vi "XNET.Cluster.Stream.Initialize.vi"(8 "error in":errorcluster, 10 "CAN Cluster":T1={"64bit Baud Rate"=125000, "Comment"="", "Name"="", "Transmit I/O Mode"=0, "64bit FD Baud Rate"=0} {"Transmit I/O Mode" items=["CAN 2.0", "CAN FD", "CAN FD+BRS"]}, 11 "database in":refnum<k21>) -> (0 "error out":errorcluster, 3 "cluster out":refnum<k21>)   [LabVIEW 2019, in "Diagnostics Addon Engine.lvlib"]
uses:
  Types/XNET.Cluster.ctl
  Diagnostics Addon Engine.lvlib
  <vilib>/xnet/xnet.llb/XNET Database Create (Cluster).vi
  <resource>/objmgr/xnet.rc
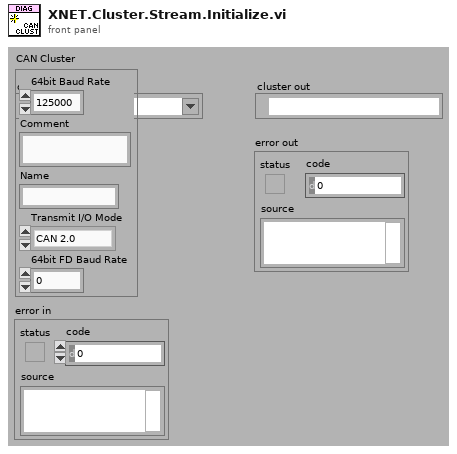
[diagram p1: front panel]
types:
  T1 = typedef "Diagnostics Addon Engine.lvlib/XNET.Cluster.ctl" = cluster{"64bit Baud Rate":u64, "Comment":string, "Name":string, "Transmit I/O Mode":u32, "64bit FD Baud Rate":u64}
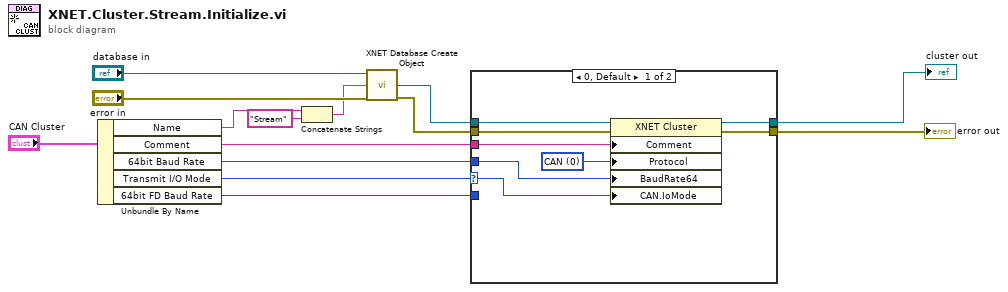
[diagram p0: block diagram]
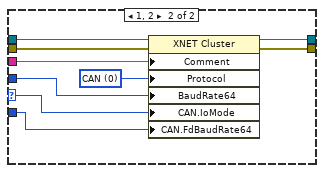
[diagram p2: hidden frame]
diagram:
  n1 = Unbundle By Name("CAN Cluster") -> ("Name"=w2:string, "Comment"=w12:string, "64bit Baud Rate"=w6:u64, "Transmit I/O Mode"=w4:u32, "64bit FD Baud Rate"=w5:u64)
  n2 = Concatenate Strings(w2, "Stream" ("string")) -> (w1:string)
  n3 = call-poly <vilib>:"XNET Database Create Object.vi"("database in"="database in", "cluster name"=w1, "error in (no error)"="error in") -> ("cluster out"=w7:refnum<k21>, "error out"=w11:errorcluster)  [unwired: 10 in, 1 out]
  n4 = case shown="0, Default" w4 {
    selector: w4 -> [w15 w24]
    tunnel: w12 -> [w21 w30]
    tunnel: w11 -> [w20 w29]
    tunnel: [w19 w28] -> w10
    tunnel: [w18 w27] -> w8
    tunnel: w7 -> [w17 w26]
    tunnel: w6 -> [w16 w25]
    tunnel: w5 -> [_ w23]
    frame 0, Default {
      w22 = u32 0 items=["CAN", "FlexRay"] ("Protocol")
      n5 = property class="XNET Cluster"(reference=w17, error in=w20, "Comment"=w21, "Protocol"=w22, "BaudRate64"=w16, "CAN.IoMode"=w15) -> (reference out=w18:refnum<k21>, error out=w19:errorcluster)
    }
    frame 1, 2 {
      w31 = u32 0 items=["CAN", "FlexRay"] ("Protocol")
      n6 = property class="XNET Cluster"(reference=w26, error in=w29, "Comment"=w30, "Protocol"=w31, "BaudRate64"=w25, "CAN.IoMode"=w24, "CAN.FdBaudRate64"=w23) -> (reference out=w27:refnum<k21>, error out=w28:errorcluster)
    }
  }
  "cluster out" <- w8
  "error out" <- w10
